vi "Globals.vi"() -> ()   [LabVIEW 2019]
panel:
  out "trigger 6 input value":bool
  in  "pxi trig 6 arbiter":T1
  in  "rxjesd.control":T2
  out "data error":bool
  in  "txjesd.control":T3
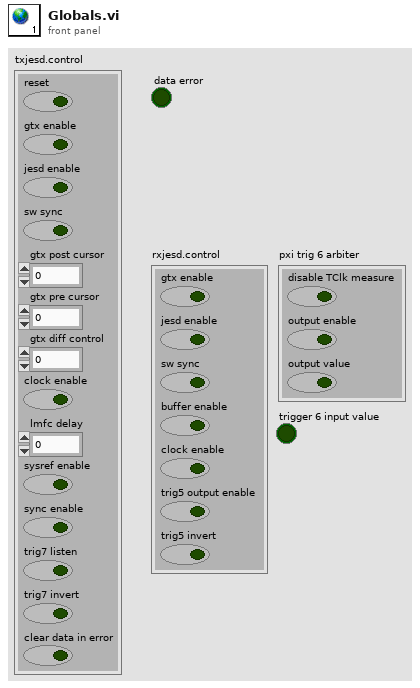
[diagram p1: front panel]
types:
  T1 = cluster{"disable TClk measure":bool, "output enable":bool, "output value":bool}
  T2 = cluster{"gtx enable":bool, "jesd enable":bool, "sw sync":bool, "buffer enable":bool, "clock enable":bool, "trig5 output enable":bool, "trig5 invert":bool}
  T3 = cluster{"reset":bool, "gtx enable":bool, "jesd enable":bool, "sw sync":bool, "gtx post cursor":fxp<+,5,5>, "gtx pre cursor":fxp<+,5,5>, "gtx diff control":fxp<+,4,4>, "clock enable":bool, "lmfc delay":fxp<+,5,5>, "sysref enable":bool, "sync enable":bool, "trig7 listen":bool, "trig7 invert":bool, "clear data in error":bool}
diagram:
